vi "Get_ADAM_Ch_names_server.vi"(1 "Channel names set":T1) -> (0 "Ch names":string[](array[string]))   [LabVIEW 2010]
uses:
  ADAM Client/Sub VIs/ADAM Controls/Channel_names.ctl
  ADAM Client/Sub VIs/ADAM Controls/Channel_State.ctl
  ADAM_Global.vi
  Sub VI's/Channel_Description_Global.vi
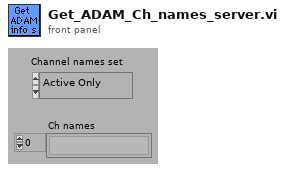
[diagram p1: front panel]
types:
  T1 = typedef "Channel_names.ctl" = enum16{"Active Only", "Active + Off", "All Channels"}
  T2 = typedef "Channel_State.ctl" = enum16{"On", "Off", "Always On", "Always Off"}
  T3 = typedef "Ch_description_ADAM.ctl" = cluster{"Ch Name":string, "Type":T4, "Function":T5, "Ch State":T2, "Calibration type":T6, "A":dbl, "B":dbl, "C":dbl, "D":dbl, "Comments":string, "Address":T7, "String":string, "Duty":u16}
  T4 = typedef "Module_type_ADAM.ctl" = enum16{"4011", "4012", "4013", "4014", "4016", "4017", "4018", "4021", "4050", "4052", "4053", "4060", "4080", "5000", "5017", "5018", "5024", "5051", "5056", "5060", "6060", "Tracker", "WEST", "GILL", "JEM", "VICI", "Vaisala", "DRUCK", "Run VI Named:", "IR2100", "PPT", "Comparator", "VIRTUAL", "Hold Value", "Read A", "Read Ch", "Coded", "Client Info", "Web Client", "X10", "Test"}
  T5 = typedef "Function_ADAM.ctl" = enum16{"Analogue Input", "Digital Input", "Event counter", "Event rate", "Analogue Output", "Digital Output", "Relay Output"}
  T6 = typedef "Calib_type_ADAM.ctl" = enum16{"Raw", "Bx + A", "Cx^2 + Bx + A", "Dx^3 + Cx^2 + Bx + A", "In Band", "Hi-Tec Q", "Hi-Tec M_dot", "Text"}
  T7 = typedef "Address.ctl" = cluster{"Main":i32, "Ch.":i32, "Sub":i32, "Port Name":string}
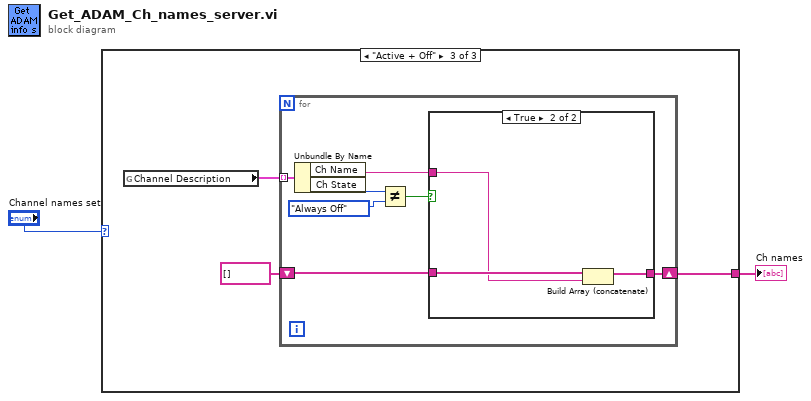
[diagram p0: block diagram]
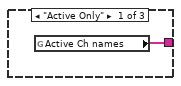
[diagram p2: hidden frame]
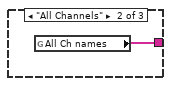
[diagram p3: hidden frame]
diagram:
  n1 = case shown="\"Active + Off\"" "Channel names set" {
    tunnel: [w3 w4 w6] -> w1
    frame "Active Only" {
      n2 = global read "ADAM_Global.vi" "Active Ch names"() -> (w3:string[])
    }
    frame "All Channels" {
      n3 = global read "ADAM_Global.vi" "All Ch names"() -> (w4:string[])
    }
    frame "Active + Off" {
      n4 = global read "Channel_Description_Global.vi" "Channel Description"() -> (w5:T3[])
      n5 = for {
        tunnel: w5 -> [w14] mode=indexing
        shift-right: [w9] -> w6
        shift-left: string[] [] -> [w10]
        n6 = Unbundle By Name(w14) -> ("Ch Name"=w8:string, "Ch State"=w13:T2)
        n7 = Not Equal?(x=w13, y=Channel_State."Always Off" ("Channel State")) -> (x != y?=w11:bool)
        n8 = case shown="True" w11 {
          tunnel: w10 -> [w15 w18]
          tunnel: [w15 w17] -> w9
          tunnel: w8 -> [_ w16]
          frame False {
          }
          frame True {
            n9 = Build Array (concatenate)(w18, w16) -> (w17:string[])
          }
        }
      }
    }
  }
  "Ch names" <- w1
